vi "Kinesis - LTS150 - Move Absolute.vi"() -> ()   [LabVIEW 2017]
uses:
  D:/X682 Camera Calibration Tester Program/data/Thorlabs.MotionControl.IntegratedStepperMotorsCLI.dll
  data/Thorlabs.MotionControl.IntegratedStepperMotorsCLI.dll
  D:/X682 Camera Calibration Tester Program/data/Thorlabs.MotionControl.Controls.dll
  data/Thorlabs.MotionControl.Controls.dll
panel:
  in  "SerialNumber":string
  in  "?":bool
  in  "Set Abs Pos":bool
  in  "MoveAbsolute":bool
  in  "Home":bool
  in  "Abs Pos":dbl
  in  "LongTravelStageControl":refnum<k24>(container)
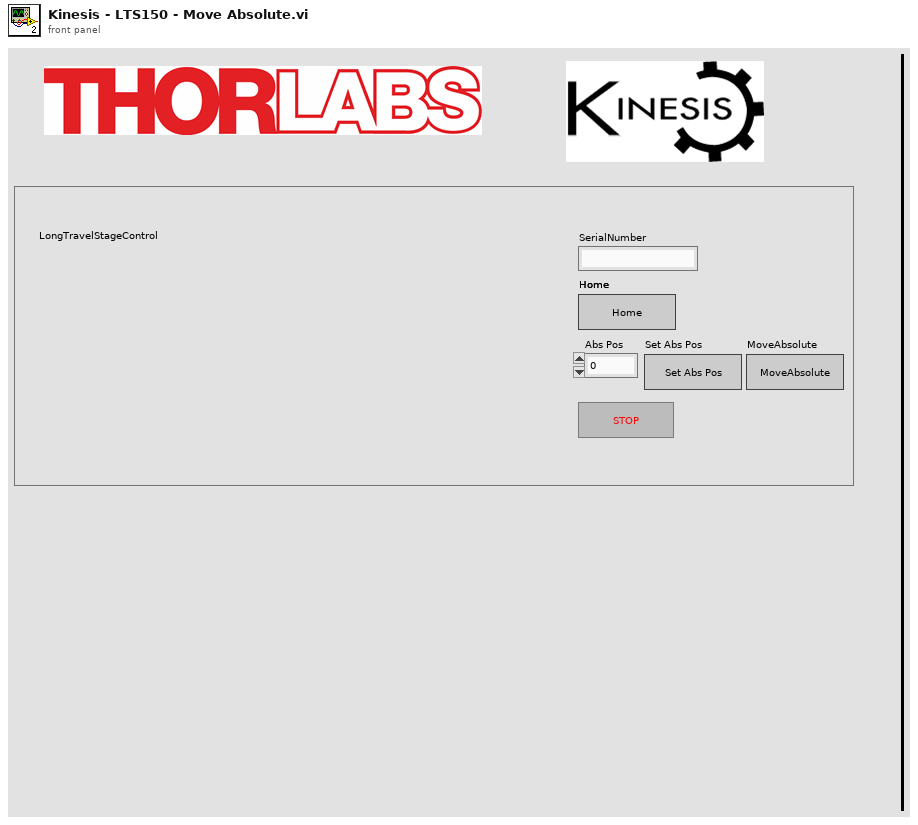
[diagram p1: front panel]
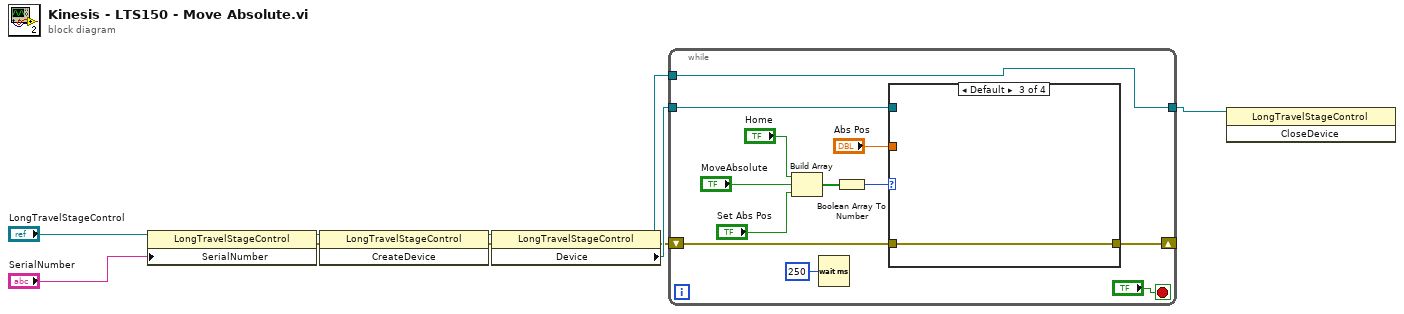
[diagram p0: block diagram]
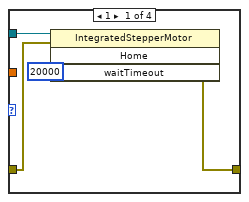
[diagram p2: hidden frame]
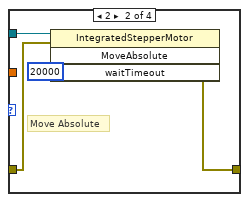
[diagram p3: hidden frame]
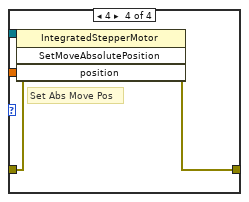
[diagram p4: hidden frame]
diagram:
  n1 = property class="LongTravelStageControl"(reference="LongTravelStageControl", "SerialNumber"="SerialNumber") -> (reference out=w9:refnum<k24>, error out=w6:errorcluster)  [unwired: 1 in]
  n2 = invoke class="LongTravelStageControl" method="CreateDevice"(reference=w9, error in=w6) -> (reference out=w8:refnum<k24>, error out=w5:errorcluster)  [unwired: 1 in, 1 out]
  n3 = property class="LongTravelStageControl"(reference=w8, error in=w5) -> (reference out=w2:refnum<k24>, error out=w4:errorcluster, "Device"=w7:refnum<k24>)
  n4 = while {
    tunnel: [w12] -> w1
    tunnel: w7 -> [w18]
    shift-right: [w15] -> _
    shift-left: w4 -> [w14]
    tunnel: w2 -> [w12]
    stop <- "?" stop-if-true
    n5 = Build Array("Home", "MoveAbsolute", "Set Abs Pos") -> (w17:bool[])
    n6 = Wait (ms)(milliseconds to wait=u32 250) -> ()  [unwired: 1 out]
    n7 = Boolean Array To Number(Boolean array=w17) -> (number=w16:u32)
    n8 = case shown="Default" w16 {
      tunnel: w18 -> [w26 w29 _ w35]
      tunnel: [w23 w27 w31 w32] -> w15
      tunnel: w14 -> [w24 w28 w31 w33]
      tunnel: "Abs Pos" -> [_ _ _ w34]
      frame 1 {
        n9 = invoke class="IntegratedStepperMotor" method="Home"(reference=w26, error in=w24, "waitTimeout"=20000) -> (error out=w23:errorcluster)  [unwired: 1 in, 3 out]
      }
      frame 2 {
        # "Move Absolute"
        n10 = invoke class="IntegratedStepperMotor" method="MoveAbsolute"(reference=w29, error in=w28, "waitTimeout"=20000) -> (error out=w27:errorcluster)  [unwired: 1 in, 3 out]
      }
      frame Default {
      }
      frame 4 {
        # "Set Abs Move Pos"
        n11 = invoke class="IntegratedStepperMotor" method="SetMoveAbsolutePosition"(reference=w35, error in=w33, "position"=w34) -> (error out=w32:errorcluster)  [unwired: 1 in, 3 out]
      }
    }
  }
  n12 = invoke class="LongTravelStageControl" method="CloseDevice"(reference=w1) -> ()  [unwired: 2 in, 3 out]
